vi "VisualizeCHROMA.vi"() -> ()   [LabVIEW 2018, in "Visualization.lvlib" / "VisualizeAcPwr.lvclass"]
uses:
  VisualizeAcPwr.lvclass
  AcPwr/MeasurmentDataCluster.ctl
  <vilib>/event_ctls.llb/usereventprio.ctl
  VisualizeBase/VisualizeBase_class/Requests/clUserEventType.ctl
  <vilib>/Utility/error.llb/Error Cluster From Error Code.vi
  <vilib>/ErrorRing/Error Ring.xnode
  VisualizeBase/VisualizeBase_class/VisualizeBase.lvclass
  <userlib>/NIST/NISTErrorLib/NISTErrorLib.lvlib
panel:
  in  "Tab Control":enum32{"Chart", "XY Graph"}(tab)
  out "Chroma":waveform(dbl)[](graph)=[{"t0"=timestamp(3657200531.6397257 s since 1904-01-01), "dt"=1.0, "Y"=[46.19]}, {"t0"=timestamp(3657200531.6397257 s since 1904-01-01), "dt"=1.0, "Y"=[2.0]}, {"t0"=timestamp(3657200531.6397257 s since 1904-01-01), "dt"=1.0, "Y"=[60.0]}]
  in  "PlotYAxis":u32[](array[numeric])=[0, 1, 0] max=1
  out "Incorrect DataType?":bool
  out "Chroma's Internal Errors/Warnings":string="No Error"
  out "Current (A)":dbl(knob) scale=0.0..15.0
  out "Voltage (V)":dbl(knob) scale=0.0..100.0
  out "XY Graph":cluster{dbl[], dbl[]}(graph)={[0.02, 0.02, 0.02, 0.02, 0.02, 0.02, 0.02, 0.02, 0.1, 0.1, 0.1, 0.1, 0.1, 0.11, 0.2, 0.2, 0.2, 0.2, 0.2, 0.2, 0.3, 0.3, 0.3, 0.3, 0.3, 0.3, 0.3, 0.37, 0.4, 0.4, 0.4, 0.4, 0.4, 0.4, 0.48, 0.5, 0.5, 0.5, 0.5, 0.5, 0.5, 0.59, 0.6, 0.6, 0.6, 0.6, 0.6, 0.6, 0.6, 0.69, 0.69, 0.69, 0.69, 0.69, 0.69, 0.71, 0.79, 0.79, 0.79, 0.79, 0.79, 0.79, 0.89, 0.89, 0.89, 0.89, 0.89, 0.89, 0.89, 1.0, 1.0, 1.0, 1.0, 1.0, 1.0, 1.0, 1.1, 1.1, 1.1, 1.09, 1.09, 1.09, 1.1, 1.19, 1.19, 1.2, 1.2, 1.2, 1.2, 1.2, 1.29, 1.29, 1.29, 1.29, 1.29, 1.29, 1.29, 1.39, 1.39, 1.39, 1.39, 1.39, 1.39, 1.39, 1.4, 1.49, 1.49, 1.49, 1.49, 1.49, 1.49, 1.57, 1.59, 1.59, 1.59, 1.59, 1.59, 1.59, 1.69, 1.69, 1.69, 1.69, 1.69, 1.69, 1.69, 1.79, 1.79, 1.79, 1.79, 1.79, 1.79, 1.79, 1.89, 1.89, 1.89, 1.89, 1.89, 1.89, 1.89, 1.99, 1.99, 1.99, 1.99, 1.99, 1.99, 2.0, 2.09, 2.09, 2.09, 2.09, 2.09, 2.09, 2.13, 2.19, 2.19, 2.19, 2.19, 2.19, 2.19, 2.29, 2.29, 2.29, 2.29, 2.29, 2.29, 2.29, 2.29, 2.39, 2.39, 2.39, 2.39, 2.39, 2.39, 2.39, 2.49, 2.49, 2.49, 2.49, 2.49, 2.49, 2.51, 2.59, 2.59, 2.59, 2.59, 2.59, 2.59, 2.69, 2.69, 2.69, 2.69, 2.69, 2.69, 2.69, 2.79, 2.79, 2.79, 2.79, 2.79, 2.79, 2.79, 2.81, 2.89, 2.89, 2.89, 2.89, 2.89, 2.89, 2.89, 2.99, 2.99, 2.99, 2.99, 2.99, 2.99, 3.0, 3.09, 3.09, 3.09, 3.09, 3.09, 3.09, 3.1, 3.19, 3.19, 3.19, 3.19, 3.19, 3.19, 3.29, 3.29, 3.29, 3.29, 3.29, 3.29, 3.29, 3.39, 3.39, 3.39, 3.39, 3.39, 3.39, 3.39, 3.39, 3.49, 3.49, 3.49, 3.49, 3.49, 3.49, 3.49, 3.5, 3.59, 3.59, 3.59, 3.59, 3.59, 3.59, 3.6, 3.69, 3.69, 3.69, 3.69, 3.69, 3.69, 3.79, 3.79, 3.79, 3.79, 3.79, 3.79, 3.79, 3.89, 3.89, 3.89, 3.89, 3.89, 3.89, 3.89, 3.99, 3.99, 3.99, 3.99, 3.99, 3.99, 3.99], [42.02, 41.83, 42.15, 41.98, 41.52, 41.47, 41.64, 41.55, 41.51, 41.49, 41.46, 41.51, 41.41, 41.39, 41.42, 41.42, 41.41, 41.4, 41.29, 41.3, 41.32, 41.33, 41.32, 41.31, 41.32, 41.21, 41.21, 41.2, 41.2, 41.21, 41.22, 41.21, 41.1, 41.1, 41.09, 41.1, 41.09, 41.11, 41.1, 40.98, 40.99, 40.98, 40.98, 40.99, 40.99, 40.98, 40.98, 40.86, 40.86, 40.88, 40.87, 40.88, 40.87, 40.87, 40.74, 40.75, 40.75, 40.75, 40.73, 40.76, 40.63, 40.63, 40.62, 40.64, 40.64, 40.61, 40.64, 40.6, 40.5, 40.46, 40.5, 40.51, 40.5, 40.51, 40.37, 40.37, 40.37, 40.37, 40.37, 40.38, 40.37, 40.36, 40.22, 40.23, 40.23, 40.24, 40.23, 40.24, 40.1, 40.09, 40.07, 40.11, 40.09, 40.09, 40.11, 39.96, 39.96, 39.95, 39.96, 39.96, 39.96, 39.94, 39.81, 39.79, 39.79, 39.81, 39.8, 39.79, 39.79, 39.81, 39.65, 39.65, 39.65, 39.65, 39.64, 39.64, 39.65, 39.48, 39.48, 39.48, 39.48, 39.47, 39.48, 39.31, 39.31, 39.3, 39.31, 39.32, 39.31, 39.31, 39.14, 39.13, 39.13, 39.14, 39.13, 39.14, 39.13, 38.95, 38.95, 38.95, 38.94, 38.95, 38.95, 38.95, 38.75, 38.75, 38.76, 38.76, 38.75, 38.75, 38.75, 38.56, 38.56, 38.56, 38.56, 38.56, 38.55, 38.34, 38.34, 38.34, 38.33, 38.33, 38.34, 38.34, 38.11, 38.11, 38.1, 38.11, 38.12, 38.1, 38.11, 38.11, 37.87, 37.86, 37.86, 37.88, 37.86, 37.88, 37.86, 37.6, 37.61, 37.61, 37.61, 37.61, 37.61, 37.62, 37.33, 37.34, 37.33, 37.34, 37.34, 37.34, 37.04, 37.04, 37.05, 37.04, 37.06, 37.05, 37.04, 36.72, 36.72, 36.71, 36.72, 36.73, 36.72, 36.71, 36.72, 36.38, 36.37, 36.39, 36.37, 36.37, 36.38, 36.37, 36.0, 36.0, 35.99, 36.0, 35.99, 36.0, 35.99, 35.59, 35.59, 35.58, 35.58, 35.58, 35.58, 35.12, 35.12, 35.12, 35.13, 35.13, 35.13, 35.12, 34.6, 34.59, 34.59, 34.59, 34.59, 34.59, 34.59, 34.6, 33.97, 33.97, 33.98, 33.97, 33.98, 33.98, 33.98, 33.26, 33.27, 33.26, 33.26, 33.26, 33.26, 33.26, 33.26, 32.38, 32.39, 32.39, 32.37, 32.37, 32.39, 32.38, 31.25, 31.24, 31.25, 31.25, 31.25, 31.25, 29.64, 29.66, 29.66, 29.67, 29.65, 29.66, 29.66, 27.14, 27.15, 27.15, 27.15, 27.14, 27.14, 27.15, 17.86, 17.84]}
  in  "PluginName":string="AcPwr.Chroma0"
  out "ErrorArray":errorcluster[](array[cluster])
  in  "QueuName":string="CHROMADCVQ"
  in  "btnStop":bool
  in  "btnReset":bool
  in  "btnClear":bool
  # "0=Left Axis and 1=Right Axis"
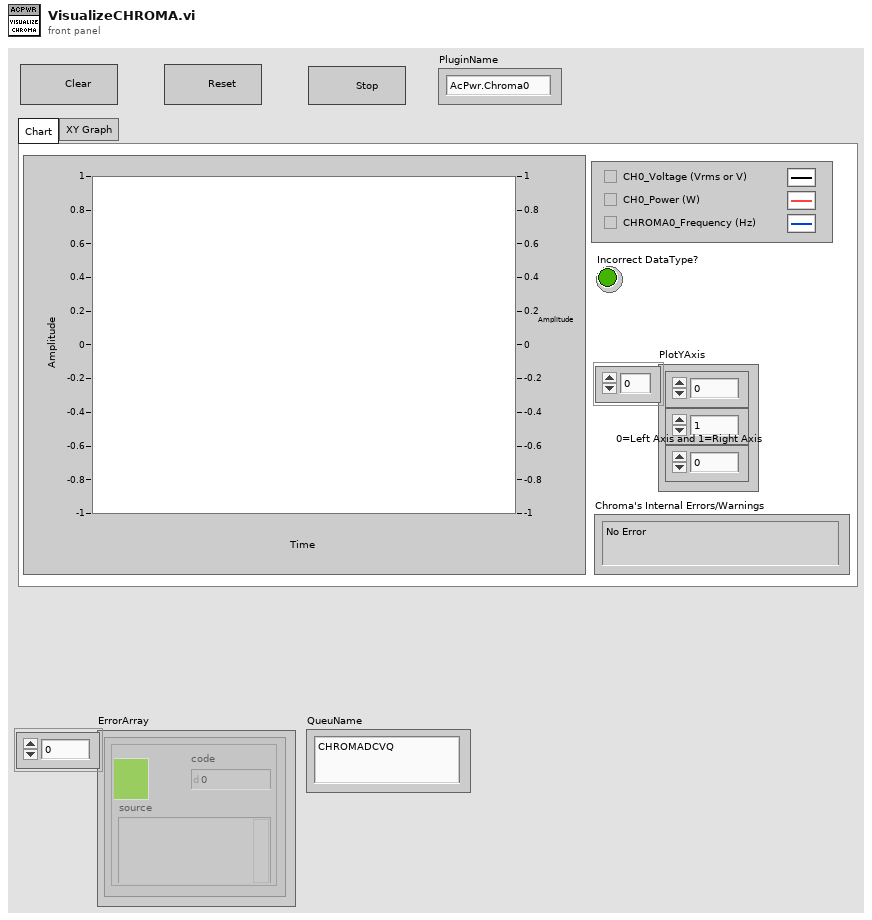
[diagram p1: front panel]
types:
  T1 = typedef "Visualization.lvlib/VisualizeBase.lvclass/clRequestEvents.ctl" = cluster{"StopRequest":refnum<user-event>, "ResetRequest":refnum<user-event>}
  T2 = typedef "clBroadcastEvents.ctl" = cluster{"DidInit":refnum<user-event>, "StatusUpdate":refnum<user-event>, "ErrorReport":refnum<user-event>, "DidStop":refnum<user-event>, "PathToINI":refnum<user-event>, "Measurements":refnum<user-event>, "LoadConfigFile":refnum<user-event>, "GetSettings":refnum<user-event>, "SetSettings":refnum<user-event>, "GetType&ID":refnum<user-event>, "GotSettings":refnum<user-event>}
  T3 = typedef "MeasurmentDataCluster.ctl" = cluster{"MeasName":string, "XML Data":string, "WaveformData":waveform(dbl)[]}
  T4 = typedef "Visualization.lvlib/VisualizeBase.lvclass/clUserEventType.ctl" = cluster{"BusIndex":i8, "Data":variant}
  T5 = typedef "usereventprio.ctl" = enum32{"high priority", "normal priority"}
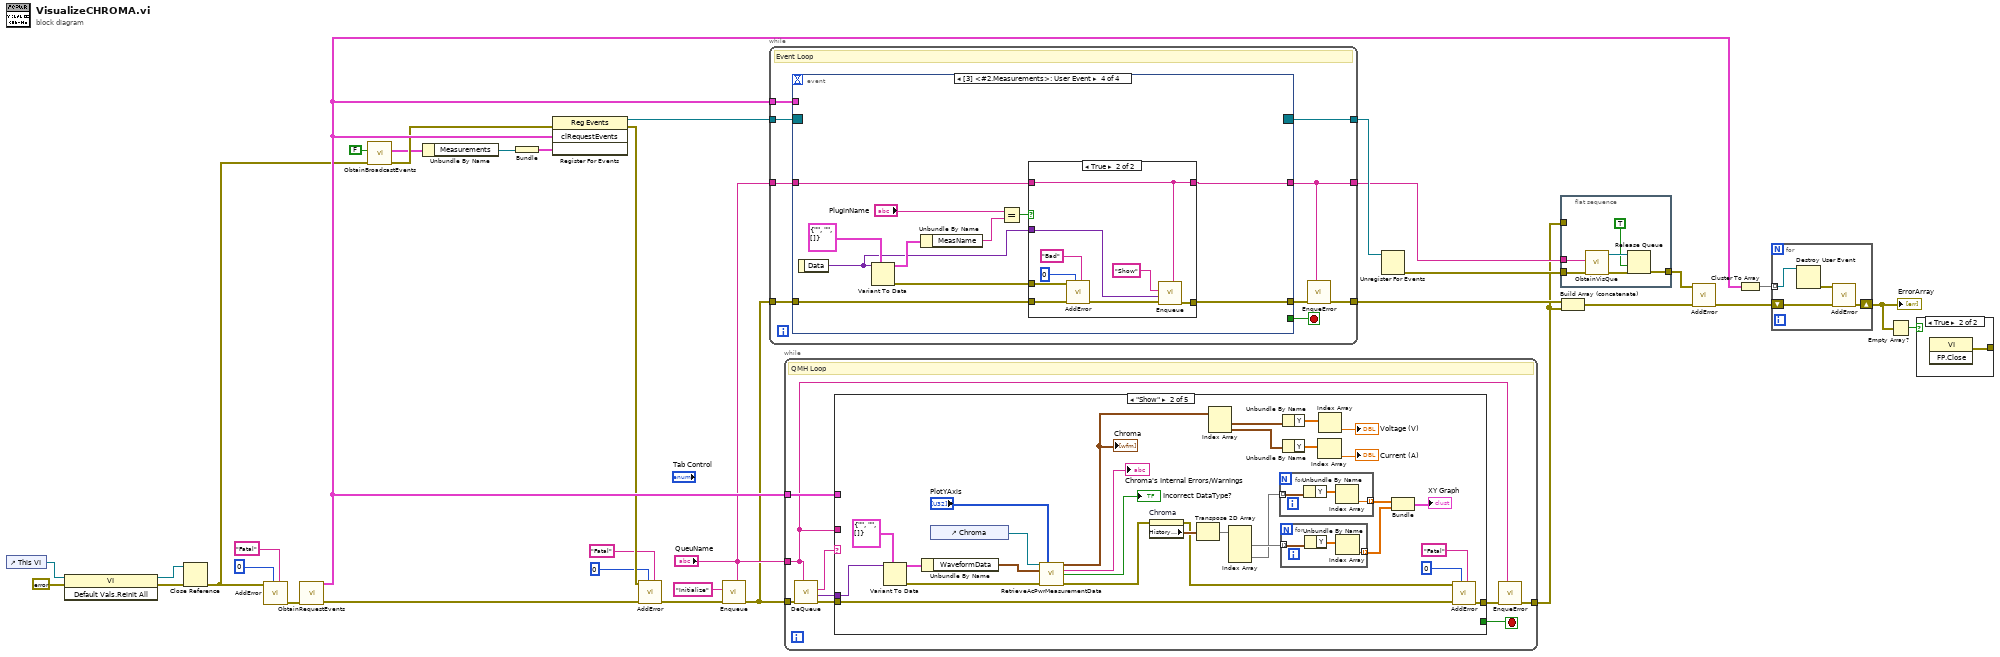
[diagram p0: block diagram]
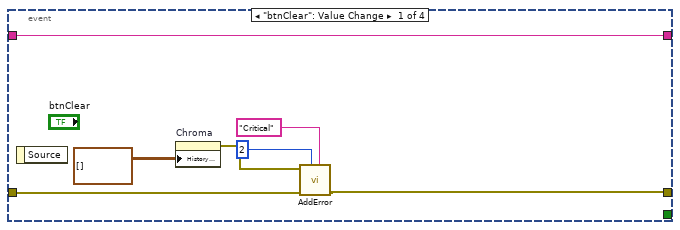
[diagram p2: hidden frame]
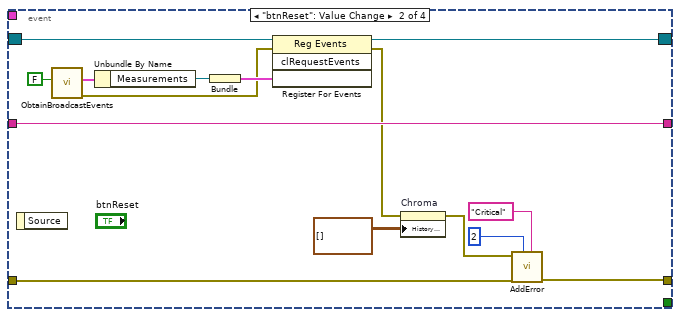
[diagram p3: hidden frame]
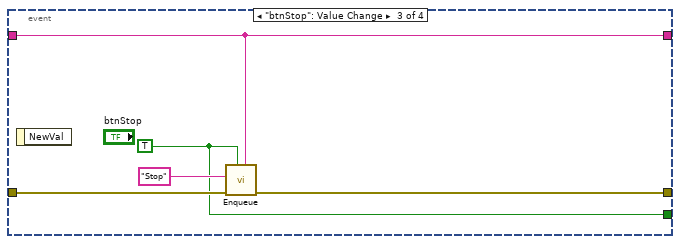
[diagram p4: hidden frame]
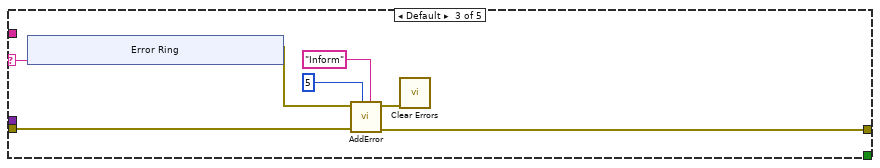
[diagram p7: hidden frame]
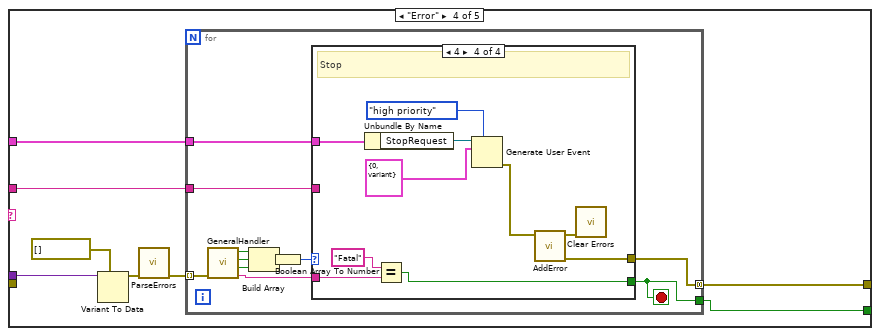
[diagram p8: hidden frame]
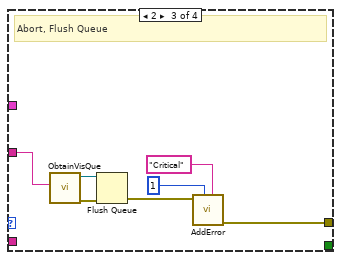
[diagram p11: hidden frame]
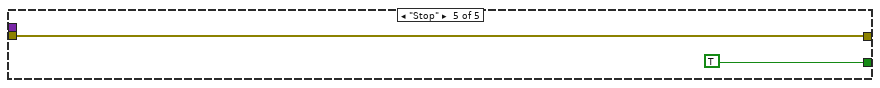
[diagram p12: hidden frame]
diagram:
  n1 = control-ref of="This VI"() -> (w20:refnum<vi>)
  n2 = invoke class="VI" method="Default Vals.Reinit All"(reference=w20, error in=errorcluster {"status"=FALSE, "code"=0, "source"=""} ("error in (no error)")) -> (reference out=w17:refnum<vi>, error out=w18:errorcluster)  [unwired: 1 in, 1 out]
  n3 = Close Reference(reference=w17, error in (no error)=w18) -> (error out=w3:errorcluster)
  n4 = call <userlib>:"AddError.vi"("Severity"="Fatal", "Priority"=u8 0, "error in (no error)"=w3) -> ("ErrorArray"=w32:errorcluster[])  [unwired: 7 in, 1 out]
  n5 = call "ObtainRequestEvents.vi"("Error"=w32) -> ("Error"=w12:errorcluster[], "clRequestEvents"=w24:T1)  [unwired: 9 in]
  n6 = call "ObtainBroadcastEvents.vi"("error in (no error)"=w3, "CreateNew? (F)"=FALSE) -> ("error out"=w4:errorcluster, "clAcPwrEvents"=w2:T2)  [unwired: 8 in]
  n7 = Unbundle By Name(w2) -> ("Measurements"=w22:refnum<user-event>)
  n8 = Bundle("Measurements"=w22) -> (w21:cluster{"Measurements":refnum<user-event>})  [unwired: 1 in]
  n9 = register-events(error in=w4, w24, w21) -> (reference out=w33:refnum<event-registration>, error out=w9:errorcluster)  [unwired: 1 in]
  n10 = call <userlib>:"AddError.vi"("Severity"="Fatal", "Priority"=u8 0, "ErrorArray"=w12, "error in (no error)"=w9) -> ("ErrorArray"=w11:errorcluster[])  [unwired: 6 in, 1 out]
  n11 = call "Enqueue.vi"("QueName"="QueuName", "Error"=w11, "Message"="Initialize") -> ("Error"=w6:errorcluster[])  [unwired: 8 in]
  n12 = while {
    tunnel: w33 -> [w43]
    tunnel: [w40] -> w29
    tunnel: [w39] -> w31
    tunnel: w24 -> [w38]
    tunnel: w6 -> [w37]
    tunnel: "QueuName" -> [w36]
    tunnel: [w35] -> w14
    stop <- w42 stop-if-true
    # "Event Loop"
    n13 = event shown="[3] <#2.Measurements>: User Event" {
      selector: w43 -> [_ w65 _ _]
      dyn-events: [_ w64 _ _] -> w39
      timeout: _ -> [_ _ _ _]
      tunnel: [_ _ w66 _] -> w42
      tunnel: [w46 w59 w67 w81] -> w41
      tunnel: w38 -> [_ _ _ _]
      tunnel: w37 -> [w47 w60 w69 w77]
      tunnel: w36 -> [w50 w61 w68 w80]
      tunnel: [w50 w61 w68 w78] -> w35
      event "btnClear": Value Change {
        n14 = event-data() -> ()  [unwired: 1 in, 1 out]
        n15 = property on="Chroma" class="WFChart (strict)"("History Data"=waveform(dbl)[][] []) -> (error out=w45:errorcluster)  [unwired: 2 in, 1 out]
        n16 = call <userlib>:"AddError.vi"("Severity"="Critical", "Priority"=u8 2, "ErrorArray"=w47, "error in (no error)"=w45) -> ("ErrorArray"=w46:errorcluster[])  [unwired: 6 in, 1 out]
      }
      event "btnReset": Value Change {
        n17 = event-data() -> ()  [unwired: 1 in, 1 out]
        n18 = call "ObtainBroadcastEvents.vi"("CreateNew? (F)"=FALSE) -> ("error out"=w53:errorcluster, "clAcPwrEvents"=w52:T2)  [unwired: 9 in]
        n19 = Unbundle By Name(w52) -> ("Measurements"=w63:refnum<user-event>)
        n20 = Bundle("Measurements"=w63) -> (w62:cluster{"Measurements":refnum<user-event>})  [unwired: 1 in]
        n21 = register-events(reference=w65, error in=w53, w62) -> (reference out=w64:refnum<event-registration>, error out=w55:errorcluster)  [unwired: 1 in]
        n22 = property on="Chroma" class="WFChart (strict)"(error in=w55, "History Data"=waveform(dbl)[][] []) -> (error out=w54:errorcluster)  [unwired: 1 in, 1 out]
        n23 = call <userlib>:"AddError.vi"("Severity"="Critical", "Priority"=u8 2, "ErrorArray"=w60, "error in (no error)"=w54) -> ("ErrorArray"=w59:errorcluster[])  [unwired: 6 in, 1 out]
      }
      event "btnStop": Value Change {
        w66 = TRUE ("Priority? (F)")
        n24 = event-data() -> ()  [unwired: 1 in, 1 out]
        n25 = call "Enqueue.vi"("QueName"=w68, "Priority? (F)"=w66, "Error"=w69, "Message"="Stop") -> ("Error"=w67:errorcluster[])  [unwired: 7 in]
      }
      event User Event {
        n26 = event-data() -> ("Data"=w71:variant)  [unwired: 1 in]
        n27 = Variant To Data(type=T3 {"MeasName"="", "XML Data"="", "WaveformData"=[]} ("MeasurmentDataCluster"), Variant=w71) -> (data=w73:T3, error out=w76:errorcluster)  [unwired: 1 in]
        n28 = Unbundle By Name(w73) -> ("MeasName"=w72:string)
        n29 = Equal?(x="PluginName", y=w72) -> (x = y?=w79:bool)
        n30 = case shown="True" w79 {
          tunnel: [w82 w91] -> w81
          tunnel: w80 -> [w83 w90]
          tunnel: w77 -> [w82 w87]
          tunnel: [w83 w90] -> w78
          tunnel: w76 -> [_ w86]
          tunnel: w71 -> [_ w84]
          frame False {
          }
          frame True {
            n31 = call <userlib>:"AddError.vi"("Severity"="Bad" ("String"), "Priority"=u8 0, "ErrorArray"=w87, "error in (no error)"=w86) -> ("ErrorArray"=w85:errorcluster[])  [unwired: 6 in, 1 out]
            n32 = call "Enqueue.vi"("QueName"=w90, "Error"=w85, "Data"=w84, "Message"="Show") -> ("Error"=w91:errorcluster[])  [unwired: 7 in]
          }
        }
      }
    }
    n33 = call "EnqueError.vi"("QueName"=w35, "Error"=w41) -> ("Error"=w40:errorcluster[])  [unwired: 9 in]
  }
  n34 = while {
    tunnel: w6 -> [w101]
    tunnel: [w95] -> w5
    tunnel: "QueuName" -> [w93]
    tunnel: w24 -> [w94]
    stop <- w96 stop-if-true
    # "QMH Loop"
    n35 = call "DeQueue.vi"("QueName"=w93, "Error"=w101) -> ("Error"=w98:errorcluster[], "Data"=w99:variant, "Message"=w100:string)  [unwired: 7 in]
    n36 = case shown="\"Show\"" w100 {
      selector: w100 -> [_ _ w144 _ _]
      tunnel: w99 -> [_ w109 _ w159 _]
      tunnel: w98 -> [w102 w129 w142 _ w188]
      tunnel: [w102 w131 w141 w155 w188] -> w97
      tunnel: [_ _ _ w154 TRUE] -> w96
      tunnel: w94 -> [_ _ _ w153 _]
      tunnel: w93 -> [_ _ _ w152 _]
      frame "Initialize" {
      }
      frame "Show" {
        n37 = Variant To Data(type=T3 {"MeasName"="", "XML Data"="", "WaveformData"=[]} ("MeasurmentDataCluster"), Variant=w109) -> (data=w107:T3, error out=w108:errorcluster)  [unwired: 1 in]
        n38 = Unbundle By Name(w107) -> ("WaveformData"=w106:waveform(dbl)[])
        n39 = control-ref of="Chroma"() -> (w130:refnum<vi>)
        n40 = call "RetrieveAcPwrMeasurementData.vi"("WaveformChartReference"=w130, "PlotYScale"="PlotYAxis", "WaveformArrayIn"=w106, "error in (no error)"=w108) -> ("WaveformArrayOut"=w116:waveform(dbl)[], "OutputString"=→"Chroma's Internal Errors/Warnings":string, "Incorrect DataType?"=→"Incorrect DataType?":bool, "error out"=w124:errorcluster)  [unwired: 7 in, 1 out]
        "Chroma" <- w116
        n41 = property on="Chroma" class="WFChart (strict)"(error in=w124) -> (error out=w104:errorcluster, "History Data"=w122:waveform(dbl)[][])  [unwired: 1 in, 1 out]
        n42 = Transpose 2D Array(2D array=w122) -> (transposed array=w123:waveform(dbl)[][])
        n43 = Index Array(array=w116) -> (element #1=w115:waveform(dbl), element #2=w114:waveform(dbl))  [unwired: 2 in]
        n44 = Index Array(array=w123) -> (element #1=w119:waveform(dbl)[], element #2=w118:waveform(dbl)[])  [unwired: 4 in]
        n45 = for {
          tunnel: w118 -> [w137] mode=indexing
          tunnel: [w135] -> w120 mode=indexing
          n46 = Unbundle By Name(w137) -> ("Y"=w136:dbl[])
          n47 = Index Array(array=w136) -> (element=w135:dbl)  [unwired: 1 in]
        }
        n48 = for {
          tunnel: w119 -> [w134] mode=indexing
          tunnel: [w132] -> w121 mode=indexing
          n49 = Unbundle By Name(w134) -> ("Y"=w133:dbl[])
          n50 = Index Array(array=w133) -> (element=w132:dbl)  [unwired: 1 in]
        }
        n51 = Unbundle By Name(w115) -> ("Y"=w113:dbl[])
        n52 = Unbundle By Name(w114) -> ("Y"=w112:dbl[])
        n53 = Index Array(array=w112) -> (element=→"Current (A)":dbl)  [unwired: 1 in]
        n54 = Index Array(array=w113) -> (element=→"Voltage (V)":dbl)  [unwired: 1 in]
        n55 = Bundle(w120, w121) -> (→"XY Graph":cluster{dbl[], dbl[]})  [unwired: 1 in]
        n56 = call <userlib>:"AddError.vi"("Severity"="Fatal" ("String"), "Priority"=u8 0, "ErrorArray"=w129, "error in (no error)"=w104) -> ("ErrorArray"=w131:errorcluster[])  [unwired: 6 in, 1 out]
      }
      frame Default {
        n57 = xnode "Error Ring"("parameter 0"=w144) -> ("error out"=w143:errorcluster)
        n58 = call <userlib>:"AddError.vi"("Severity"="Inform" ("String"), "Priority"=u8 5, "ErrorArray"=w142, "error in (no error)"=w143) -> ("ErrorArray"=w141:errorcluster[], "error out"=w140:errorcluster)  [unwired: 6 in]
        n59 = call <vilib>:"Clear Errors.vi"("error in (no error)"=w140) -> ()  [unwired: 5 in, 2 out]
      }
      frame "Error" {
        n60 = Variant To Data(type=errorcluster[] [], Variant=w159) -> (data=w157:errorcluster[])  [unwired: 1 in, 1 out]
        n61 = call <userlib>:"ParseErrors.vi"("ErrorArray"=w157) -> ("ErrorArray"=w156:errorcluster[])  [unwired: 8 in, 2 out]
        n62 = for {
          tunnel: w156 -> [w170] mode=indexing
          tunnel: [w164] -> w155 mode=concatenating
          tunnel: [w162] -> w154
          tunnel: w153 -> [w161]
          tunnel: w152 -> [w160]
          stop <- w162 stop-if-true
          n63 = call <userlib>:"GeneralHandler.vi"("error in (no error)"=w170) -> ("Severity"=w163:string, "Stop"=w167:bool, "Abort"=w168:bool, "Continue"=w169:bool)  [unwired: 7 in]
          n64 = Build Array(w169, w168, w167) -> (w166:bool[])
          n65 = Boolean Array To Number(Boolean array=w166) -> (number=w165:u32)
          n66 = case shown="4" w165 {
            tunnel: [_ _ w175 w186] -> w164
            tunnel: w163 -> [_ _ _ w181]
            tunnel: [_ _ _ w179] -> w162
            tunnel: w161 -> [_ _ _ w178]
            tunnel: w160 -> [_ _ w171 _]
            frame 0, Default {
              # "No Dialog"
            }
            frame 1 {
              # "Continue"
            }
            frame 2 {
              # "Abort, Flush Queue"
              n67 = call "ObtainVisQue.vi"("QueName"=w171) -> ("error out"=w177:errorcluster, "queue out"=w176:refnum<queue>)  [unwired: 9 in]
              n68 = Flush Queue(queue=w176, error in (no error)=w177) -> (error out=w174:errorcluster)  [unwired: 2 out]
              n69 = call <userlib>:"AddError.vi"("Severity"="Critical" ("String"), "Priority"=u8 1, "error in (no error)"=w174) -> ("ErrorArray"=w175:errorcluster[])  [unwired: 7 in, 1 out]
            }
            frame 4 {
              # "Stop"
              n70 = Unbundle By Name(w178) -> ("StopRequest"=w187:refnum<user-event>)
              n71 = Equal?(x="Fatal", y=w181) -> (x = y?=w179:bool)
              n72 = Generate User Event(priority (normal)=usereventprio."high priority", user event=w187, event data cluster=T4 {"BusIndex"=0, "Data"=variant} ("event data")) -> (error out=w185:errorcluster)  [unwired: 1 in, 1 out]
              n73 = call <userlib>:"AddError.vi"("error in (no error)"=w185) -> ("ErrorArray"=w186:errorcluster[], "error out"=w182:errorcluster)  [unwired: 9 in]
              n74 = call <vilib>:"Clear Errors.vi"("error in (no error)"=w182) -> ()  [unwired: 5 in, 2 out]
            }
          }
        }
      }
      frame "Stop" {
      }
    }
    n75 = call "EnqueError.vi"("QueName"=w93, "Error"=w97) -> ("Error"=w95:errorcluster[])  [unwired: 9 in]
  }
  n76 = Unregister For Events(event registration refnum=w31) -> (error out=w28:errorcluster)  [unwired: 1 in]
  n77 = flat-sequence {
    tunnel: w28 -> [w195]
    tunnel: [w192] -> w26
    tunnel: w14 -> [w191]
    tunnel: w5 -> [_]
    frame #0 {
      n78 = call "ObtainVisQue.vi"("error in (no error)"=w195, "QueName"=w191) -> ("error out"=w194:errorcluster, "queue out"=w193:refnum<queue>)  [unwired: 8 in]
      n79 = Release Queue(queue=w193, force destroy? (F)=TRUE, error in (no error)=w194) -> (error out=w192:errorcluster)  [unwired: 2 out]
    }
  }
  n80 = Build Array (concatenate)(w29, w5) -> (w27:errorcluster[])
  n81 = call <userlib>:"AddError.vi"("ErrorArray"=w27, "error in (no error)"=w26) -> ("ErrorArray"=w25:errorcluster[])  [unwired: 8 in, 1 out]
  n82 = Cluster To Array(cluster=w24) -> (array=w30:refnum<user-event>[])
  n83 = for {
    tunnel: w30 -> [w199] mode=indexing
    shift-right: [w198] -> w16
    shift-left: w25 -> [w197]
    n84 = Destroy User Event(user event=w199) -> (error out=w196:errorcluster)  [unwired: 1 in]
    n85 = call <userlib>:"AddError.vi"("ErrorArray"=w197, "error in (no error)"=w196) -> ("ErrorArray"=w198:errorcluster[])  [unwired: 8 in, 1 out]
  }
  "ErrorArray" <- w16
  n86 = Empty Array?(array=w16) -> (empty?=w23:bool)
  n87 = case shown="True" w23 {
    tunnel: [_ w200] -> _
    frame False {
    }
    frame True {
      n88 = invoke class="VI" method="FP.Close"() -> (error out=w200:errorcluster)  [unwired: 3 in, 2 out]
    }
  }
